vi "TransformDataTypeHelper.vi"   [LabVIEW 2017]
uses:
  Shared/PathFileData.ctl
  Shared/RobotNeededPathData.ctl
types:
  T1 = typedef "PathFileData.ctl" = cluster{"RobotNeeded":T2, "Meta":cluster{"Path (px)":cluster{i32, i32}[], "RobotWidth":dbl, "RobotLength":dbl, "CenterOfRotYOffset":dbl, "Roundedness":dbl, "StartingPositionPreset":u32, "PathName":string}}
  T2 = typedef "RobotNeededPathData.ctl" = cluster{"Path":cluster{dbl, dbl}[], "MaxVel":dbl, "MaxAccel":dbl, "Backwards?":bool, "PointSpacing":dbl, "LookaheadDist":dbl, "Speed/Curve":dbl, "SlowDistanceAtEnd":dbl, "SlowSpeed":dbl, "MaxDeAccel":dbl}
  T3 = cluster{"RobotNeeded":cluster{"Path":cluster{dbl, dbl}[], "MaxVel":dbl, "MaxAccel":dbl, "Backwards?":bool, "PointSpacing":dbl, "LookaheadDist":dbl, "Speed/Curve":dbl, "SlowDistanceAtEnd":dbl, "SlowSpeed":dbl}, "Meta":cluster{"Path (px)":cluster{i32, i32}[], "RobotWidth":dbl, "RobotLength":dbl, "CenterOfRotYOffset":dbl, "Roundedness":dbl, "StartingPositionPreset":u32, "PathName":string}}
  T4 = cluster{"Path":cluster{dbl, dbl}[], "MaxVel":dbl, "MaxAccel":dbl, "Backwards?":bool, "PointSpacing":dbl, "LookaheadDist":dbl, "Speed/Curve":dbl, "SlowDistanceAtEnd":dbl, "SlowSpeed":dbl}
  T5 = cluster{"Path (px)":cluster{i32, i32}[], "RobotWidth":dbl, "RobotLength":dbl, "CenterOfRotYOffset":dbl, "Roundedness":dbl, "StartingPositionPreset":u32, "PathName":string}
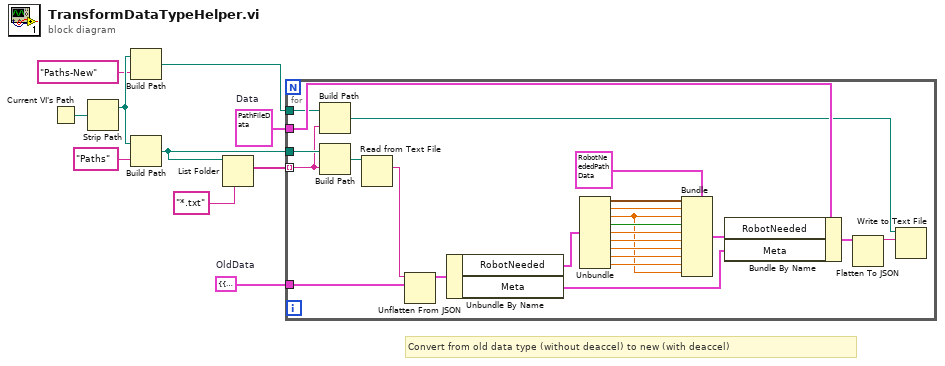
[diagram p0: block diagram]
diagram:
  w4 = T1 {"RobotNeeded"={"Path"=[], "MaxVel"=0.0, "MaxAccel"=0.0, "Backwards?"=FALSE, "PointSpacing"=0.0, "LookaheadDist"=0.0, "Speed/Curve"=1.8, "SlowDistanceAtEnd"=12.0, "SlowSpeed"=15.0, "MaxDeAccel"=0.0}, "Meta"={"Path (px)"=[], "RobotWidth"=0.0, "RobotLength"=0.0, "CenterOfRotYOffset"=0.0, "Roundedness"=0.0, "StartingPositionPreset"=0, "PathName"=""}}  # Data
  w9 = T3 {"RobotNeeded"={"Path"=[], "MaxVel"=0.0, "MaxAccel"=0.0, "Backwards?"=FALSE, "PointSpacing"=0.0, "LookaheadDist"=0.0, "Speed/Curve"=1.8, "SlowDistanceAtEnd"=12.0, "SlowSpeed"=15.0}, "Meta"={"Path (px)"=[], "RobotWidth"=0.0, "RobotLength"=0.0, "CenterOfRotYOffset"=0.0, "Roundedness"=0.0, "StartingPositionPreset"=2, "PathName"=""}}  # OldData
  # "Convert from old data type (without deaccel) to new (with deaccel)"
  n1 = Current VI's Path() -> (path=w8:path)
  n2 = Strip Path(path=w8) -> (stripped path=w3:path)  [unwired: 1 out]
  n3 = Build Path(base path=w3, name or relative path="Paths-New") -> (appended path=w1:path)
  n4 = Build Path(base path=w3, name or relative path="Paths") -> (appended path=w5:path)
  n5 = List Folder(path=w5, pattern="*.txt") -> (filenames=w6:string[])  [unwired: 2 in, 3 out]
  n6 = for {
    tunnel: w9 -> [w34]
    tunnel: w5 -> [w31]
    tunnel: w6 -> [w12] mode=indexing
    tunnel: w4 -> [w29]
    tunnel: w1 -> [w13]
    n7 = Build Path(base path=w13, name or relative path=w12) -> (appended path=w11:path)
    n8 = Build Path(base path=w31, name or relative path=w12) -> (appended path=w32:path)
    n9 = Read from Text File(file (use dialog)=w32) -> (text=w30:string)  [unwired: 3 in, 3 out]
    n10 = Unflatten From JSON(JSON string=w30, type and defaults=w34) -> (value=w33:T3)  [unwired: 5 in, 1 out]
    n11 = Unbundle By Name(w33) -> ("RobotNeeded"=w27:T4, "Meta"=w28:T5)
    n12 = Unbundle(w27) -> ("Path"=w25:cluster{dbl, dbl}[], "MaxVel"=w24:dbl, "MaxAccel"=w17:dbl, "Backwards?"=w23:bool, "PointSpacing"=w22:dbl, "LookaheadDist"=w21:dbl, "Speed/Curve"=w20:dbl, "SlowDistanceAtEnd"=w19:dbl, "SlowSpeed"=w18:dbl)
    n13 = Bundle(cluster=T2 {"Path"=[], "MaxVel"=0.0, "MaxAccel"=0.0, "Backwards?"=FALSE, "PointSpacing"=0.0, "LookaheadDist"=0.0, "Speed/Curve"=1.8, "SlowDistanceAtEnd"=12.0, "SlowSpeed"=15.0, "MaxDeAccel"=0.0} ("RobotNeeded"), "Path"=w25, "MaxVel"=w24, "MaxAccel"=w17, "Backwards?"=w23, "PointSpacing"=w22, "LookaheadDist"=w21, "Speed/Curve"=w20, "SlowDistanceAtEnd"=w19, "SlowSpeed"=w18, "MaxDeAccel"=w17) -> (w16:T2)
    n14 = Bundle By Name(cluster=w29, "RobotNeeded"=w16, "Meta"=w28) -> (w15:T1)
    n15 = Flatten To JSON(anything=w15) -> (JSON string=w14:string)  [unwired: 2 in, 1 out]
    n16 = Write to Text File(file (use dialog)=w11, text=w14) -> ()  [unwired: 2 in, 3 out]
  }
